vi "Reset.vi"(8 "Error in (no error)":errorcluster, 11 "VISA resource":refnum<visa-resource-name>) -> (0 "Error out":errorcluster, 3 "Dup VISA resource":refnum<visa-resource-name>)   [LabVIEW 2010]
doc: "Copyright (c) 2012 Metrolab Technology SA, Plan-les-Ouates, Geneva, Switzerland\nReset the instrument to startup settings:\n- Averaging: 1\n- Acquisition buffer: empty\n- Trigger source: Immediate\n- Trigger count: 1\n- Trigger timer: 100 ms\n- Range: Auto\n- Calibration state: On\n- Units: Tesla\n- Format: ASCII\n- Status: cleared, enable regiters reset"
panel:
  # "RESET"
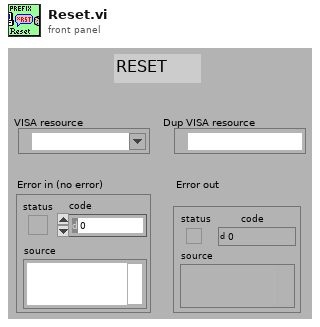
[diagram p1: front panel]
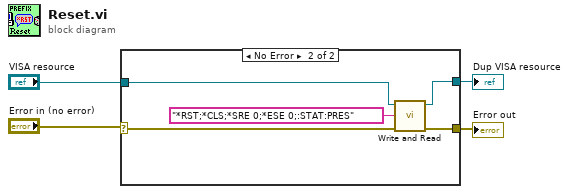
[diagram p0: block diagram]
diagram:
  n1 = case shown="No Error" "Error in (no error)" {
    selector: "Error in (no error)" -> [w6 w10]
    tunnel: [w5 w9] -> w1
    tunnel: [w6 w11] -> w4
    tunnel: "VISA resource" -> [w5 w7]
    frame Error {
    }
    frame No Error {
      n2 = call "Write and Read.vi"("Error in (no error)"=w10, "Command"="*RST;*CLS;*SRE 0;*ESE 0;:STAT:PRES" ("Reset Command"), "VISA resource"=w7) -> ("Error out"=w11:errorcluster, "Dup VISA resource"=w9:refnum<visa-resource-name>)  [unwired: 4 in, 3 out]
    }
  }
  "Error out" <- w4
  "Dup VISA resource" <- w1
